vi "tHD_STA.vi"(0 "waveform":waveform(dbl), 1 "Add Points":dbl=10.0, 2 "Index":dbl[](array[numeric]), 3 "VDDA":dbl=2.5, 4 "index 2":i32=41, 5 "index":i32=22, 7 "for Reg Ack bit":i32) -> (11 "Data Binary":bool[](array[boolean])=[TRUE, TRUE, TRUE, TRUE, TRUE, FALSE, FALSE, TRUE, TRUE, TRUE, FALSE, TRUE], 12 "Data":u32=2975 format="%.0x", 13 "Data ACK":bool, 14 "Address":u32=2975 format="%.0x", 15 "Address ACK":bool, 16 "Address Binary":bool[](array[boolean])=[TRUE, TRUE, TRUE, TRUE, TRUE, FALSE, FALSE, TRUE, TRUE, TRUE, FALSE, TRUE], 17 "Reg Address":u32=2975 format="%.0x", 18 "Reg Address ACK":bool, 19 "Reg Address  Binary":bool[](array[boolean])=[TRUE, TRUE, TRUE, TRUE, TRUE, FALSE, FALSE, TRUE, TRUE, TRUE, FALSE, TRUE])   [LabVIEW 2019]
panel:
  out "VDDA 2":dbl=2.5
  out "Data 3":dbl[](array[numeric])
  out "Reg Address":dbl[](array[numeric])
  out "Address":dbl[](array[numeric])
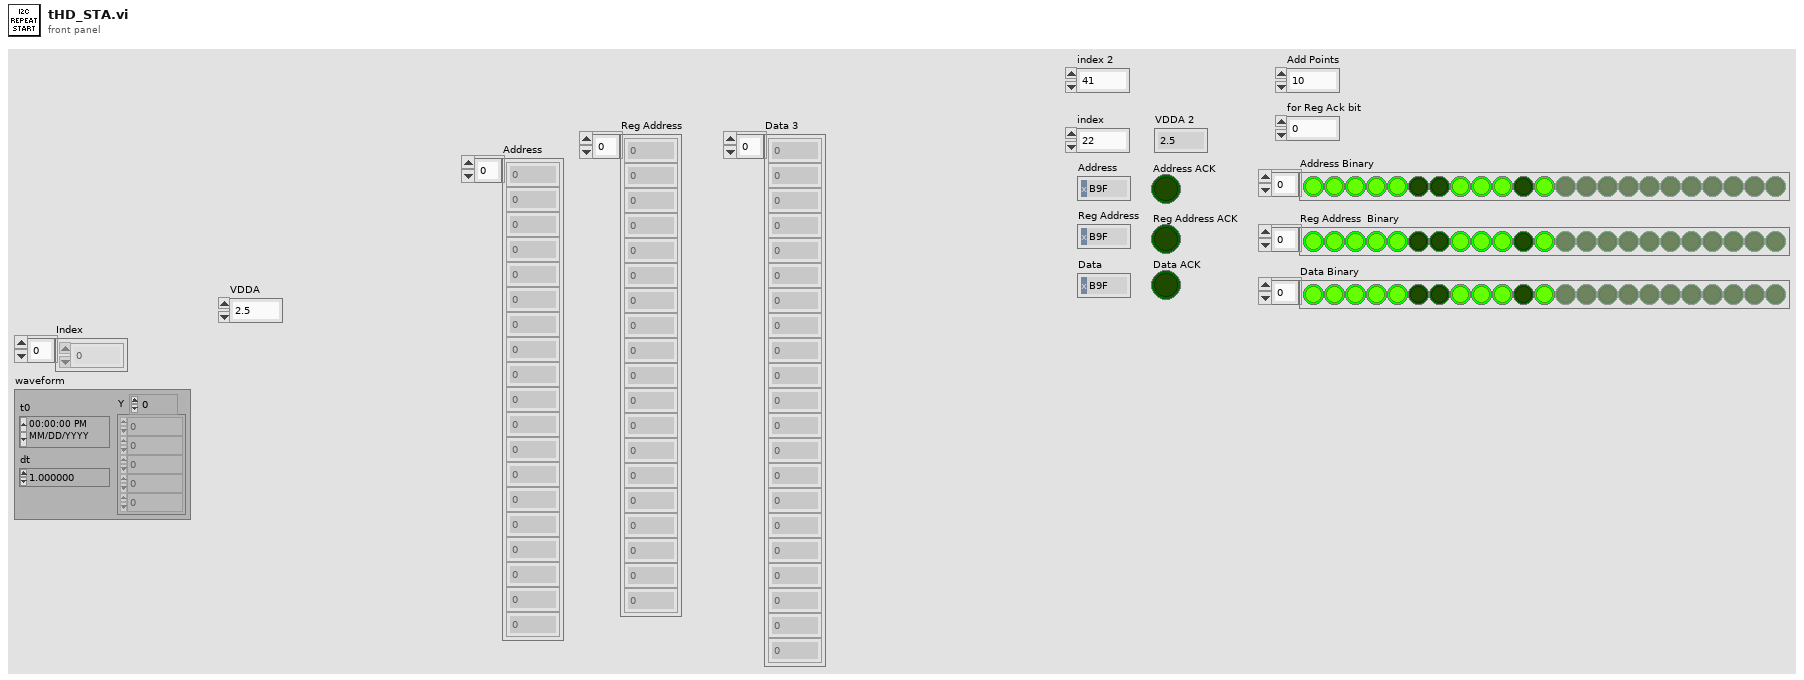
[diagram p1: front panel]
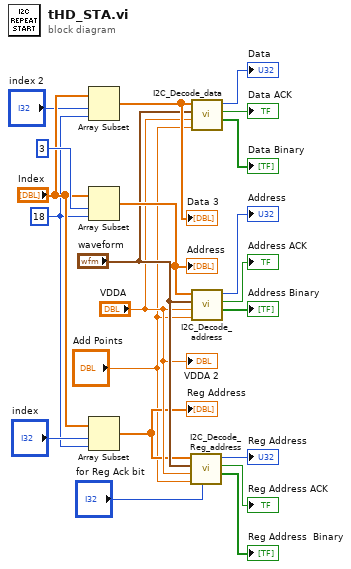
[diagram p0: block diagram]
diagram:
  w10 = 18 ("length")
  n1 = Array Subset(array="Index", index="index 2", length=w10) -> (w12:dbl[])
  "Data 3" <- w12
  n2 = Array Subset(array="Index", index=3, length=w10) -> (w19:dbl[])
  "Address" <- w19
  n3 = Array Subset(array="Index", index="index", length=w10) -> (w3:dbl[])
  "Reg Address" <- w3
  n4 = call "I2C_Decode_Reg_address.vi"("for Ack bit"="for Reg Ack bit", "Add Points"="Add Points", "VDDA"="VDDA", "waveform"="waveform", "Index"=w3) -> ("Reg Address Binary"=→"Reg Address  Binary":bool[], "Reg Address ACK"=→"Reg Address ACK":bool, "Reg Address"=→"Reg Address":u32)  [unwired: 4 in]
  n5 = call "I2C_Decode_data.vi"("Add points"="Add Points", "VDDA 3"="VDDA", "waveform"="waveform", "Index"=w12) -> ("Data Binary"=→"Data Binary":bool[], "Data ACK"=→"Data ACK":bool, "Data"=→"Data":u32)  [unwired: 5 in]
  n6 = call "I2C_Decode_address.vi"("Add points"="Add Points", "VDDA"="VDDA", "waveform"="waveform", "Index"=w19) -> ("Address Binary"=→"Address Binary":bool[], "Address ACK"=→"Address ACK":bool, "Address"=→"Address":u32)  [unwired: 5 in]
  "VDDA 2" <- "VDDA"
